vi "ScriptWrite.vi"(0 "Marker shape":string, 1 "Traces.txt":string, 2 "PNG file name":string, 5 "Marker size":i32, 7 "Traces colors string (RGB)":string[](array[string]), 9 "PDF file path":path, 11 "Script.m path":path, 12 "TracesRead error":errorcluster) -> (6 "Script.m":string, 14 "ScriptWrite error out":errorcluster)   [LabVIEW 2023]
panel:
  in  "User interface":T1(tab)
  in  "User entries":enum32{""}(tab)
  in  "Customization":enum32{"Customization"}(tab)
  in  "Colors":enum32{"Colors"}(tab)
  in  "Size":enum32{"Size"}(tab)
  in  "Loop FOR 1":enum32{"Loop FOR 1"}(tab)
  in  "Arrays":enum32{"Arrays"}(tab)
  in  "Script.m":enum32{"Script.m"}(tab)
  out "Colors string":string
  in  "Extract.c output string scan":enum32{"Extract.c output string scan"}(tab)
  in  "T: tt1 tt2 tt3 ...":enum32{"T: tt1 tt2 tt3 ..."}(tab)
  in  "C: cc":enum32{"C: cc"}(tab)
  in  "Loop FOR 2":enum32{"Loop FOR 2"}(tab)
  in  "LabVIEW":enum32{"LabVIEW"}(tab)
  in  "MATLAB":enum32{"MATLAB"}(tab)
  in  "C":enum32{"C"}(tab)
  in  "MATLAB":enum32{"MATLAB"}(tab)
  in  "C":enum32{"C"}(tab)
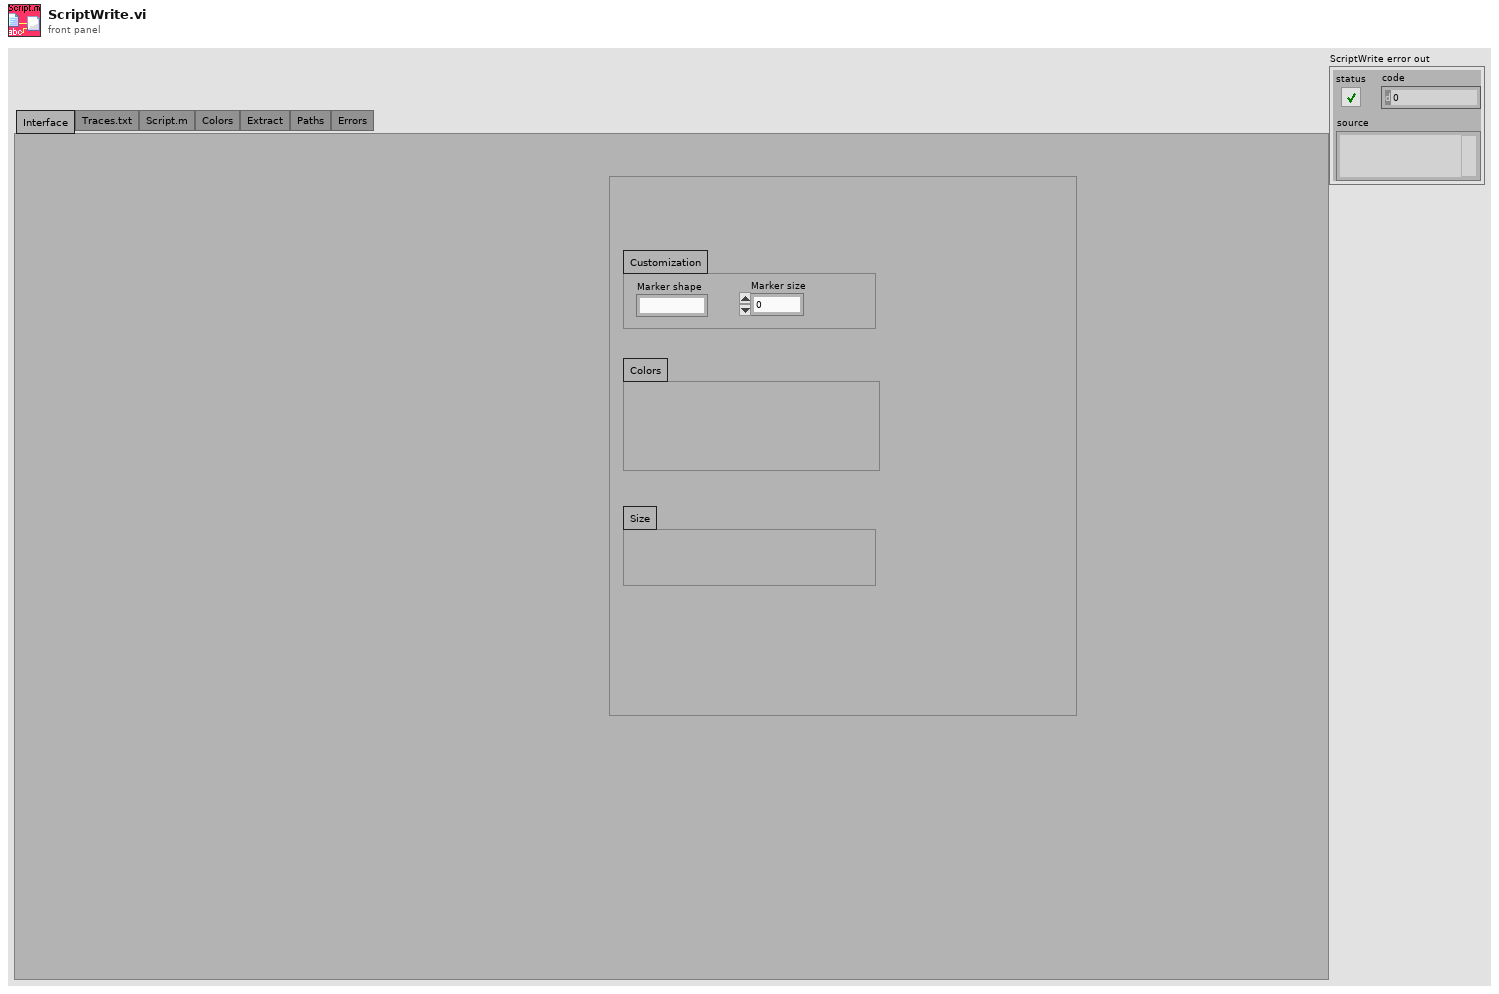
[diagram p1: front panel]
types:
  T1 = enum32{"Interface", "Traces.txt", "Script.m", "Colors", "Extract", "Paths", "Errors"}
  T2 = enum16{"open", "replace", "create", "open or create", "replace or create", "replace or create with confirmation"}
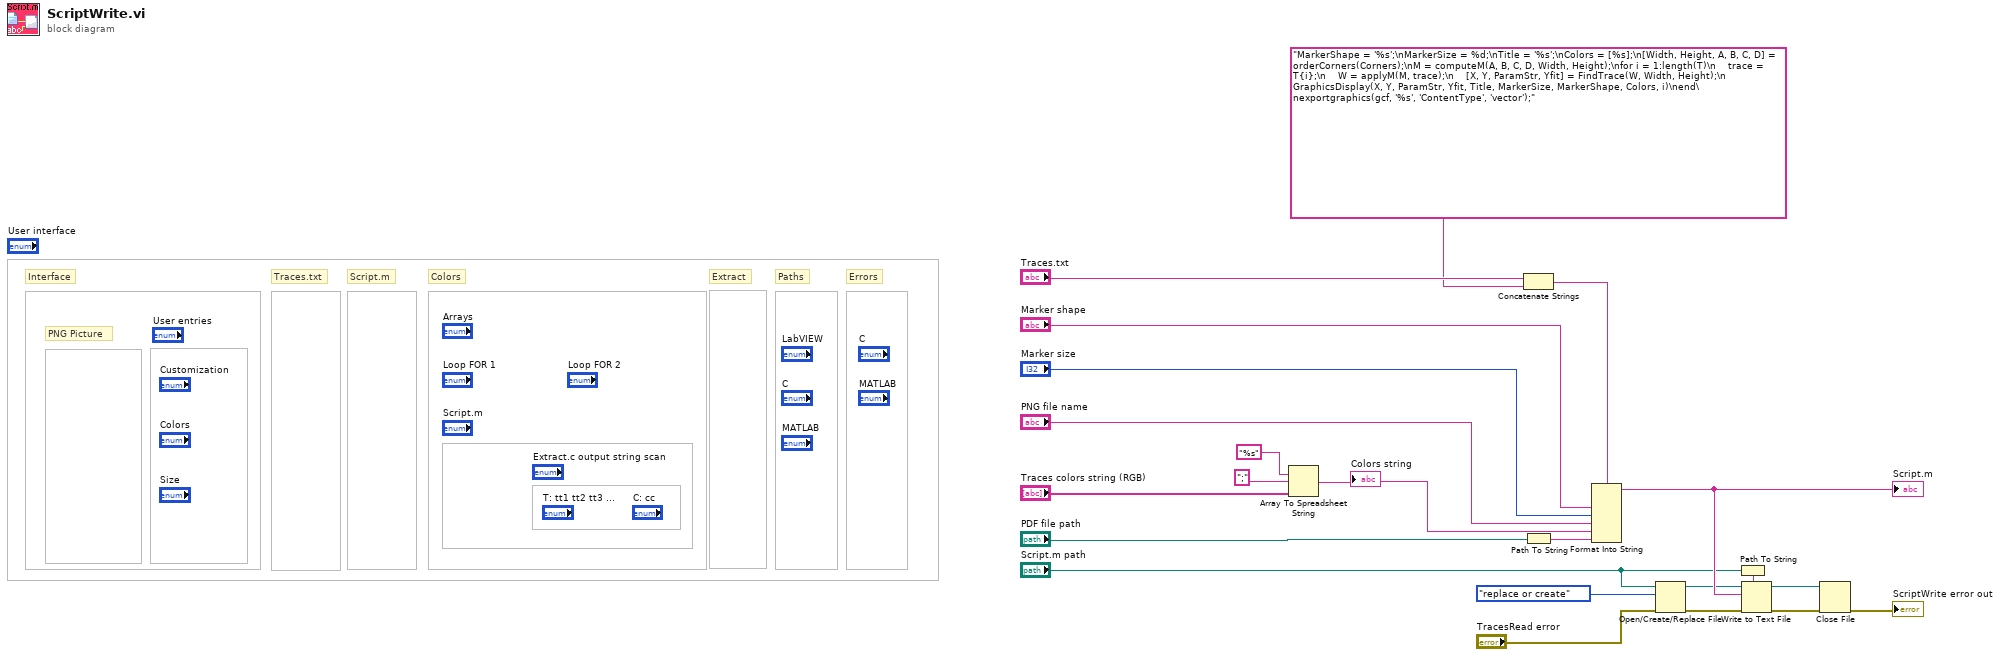
[diagram p0: block diagram]
diagram:
  # "PNG Picture"
  # "Errors"
  # "Paths"
  # "Extract"
  # "Colors"
  # "Script.m"
  # "Traces.txt"
  # "Interface"
  n1 = Array To Spreadsheet String(delimiter (Tab)=";", array="Traces colors string (RGB)", 3:"%s" ("format string")) -> (spreadsheet string=w7:string)
  "Colors string" <- w7
  n2 = Concatenate Strings("Traces.txt", "MarkerShape = '%s';\nMarkerSize = %d;\nTitle = '%s';\nColors = [%s];\n[Width, Height, A, B, C, D] = orderCorners(Corners);\nM = computeM(A, B, C, D, Width, Height);\nfor i = 1:length(T)\n    trace = T{i};\n    W = applyM(M, trace);\n    [X, Y, ParamStr, Yfit] = FindTrace(W, Width, Height);\n    GraphicsDisplay(X, Y, ParamStr, Yfit, Title, MarkerSize, MarkerShape, Colors, i)\nend\nexportgraphics(gcf, '%s', 'ContentType', 'vector');" ("initial string")) -> (w10:string)
  n3 = Path To String(path="PDF file path") -> (string=w6:string)
  n4 = Format Into String(format string=w10, "Marker shape", "Marker size", "PNG file name", w7, w6) -> (resulting string=w22:string)  [unwired: 2 in, 1 out]
  "Script.m" <- w22
  n5 = Open/Create/Replace File(file path (use dialog)="Script.m path", error in="TracesRead error", operation (0:open)=T2."replace or create") -> (refnum out=w21:refnum<file>, error out=w19:errorcluster)  [unwired: 3 in, 1 out]
  n6 = Path To String(path="Script.m path") -> (string=w16:string)
  n7 = Write to Text File(prompt (Choose or enter file path)=w16, file (use dialog)=w21, text=w22, error in=w19) -> (refnum out=w17:refnum<file>, error out=w18:errorcluster)  [unwired: 1 out]
  n8 = Close File(refnum=w17, error in=w18) -> (error out=→"ScriptWrite error out":errorcluster)  [unwired: 1 out]
